vi "SPARK Get Encoder Status.vi"   [LabVIEW 2023]
doc: "Get the periodic status of the primary encoder of the SPARK."
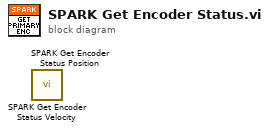
[diagram p0: block diagram]
diagram:
  n1 = call "SPARK Get Encoder Status Velocity.vi"() -> ()  [unwired: 8 in, 4 out]
  n2 = call "SPARK Get Encoder Status Position.vi"() -> ()  [unwired: 8 in, 4 out]
